vi "Request Data JSON.vi"(8 "error in (no error)":errorcluster, 11 "GetInputMute in":refnum<class "GetInputMute.lvclass">) -> (0 "error out":errorcluster, 2 "Request Data JSON":string, 3 "GetInputMute out":refnum<class "GetInputMute.lvclass">)   [LabVIEW 2020, in "obs-websocket.lvlib" / "GetInputMute.lvclass"]
uses:
  GetInputMute.lvclass
  GetInputMute.lvclass/GetInputMute.ctl
  9a249a72-5178-42ea-b031-a8aa7555a28c.vi
  <vilib>/JDP Science/JSONtext/Variant to JSON Text.vi
  <vilib>/JDP Science/JSONtext/LVClass Serializer/JSONtext LVClass Serializer.lvclass
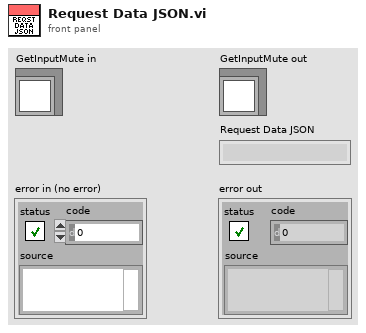
[diagram p1: front panel]
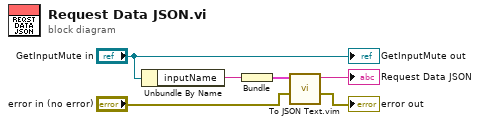
[diagram p0: block diagram]
diagram:
  n1 = Unbundle By Name("GetInputMute in") -> ("inputName"=w5:string)
  n2 = Bundle("inputName"=w5) -> (w4:cluster{"inputName":string})  [unwired: 1 in]
  n3 = call "To JSON Text.vim"("error in (no error)"="error in (no error)", "Anything"=w4) -> ("error out"=→"error out":errorcluster, "<JSON>"=→"Request Data JSON":string)  [unwired: 8 in]
  "GetInputMute out" <- "GetInputMute in"
